vi "Write ID.vi"(8 "id":u32, 11 "Channel Message in":refnum<class "Channel Message.lvclass">) -> (3 "Channel Message out":refnum<class "Channel Message.lvclass">)   [LabVIEW 2017, in "Channel Message.lvclass"]
doc: "Writes the ID for this message. This is done automatically when the message is written into the Messenger Channel."
uses:
  <vilib>/ChannelSupport/Channel Message/Channel Message.lvclass
  <vilib>/ChannelSupport/Channel Message/Channel Message.lvclass/Channel Message.ctl
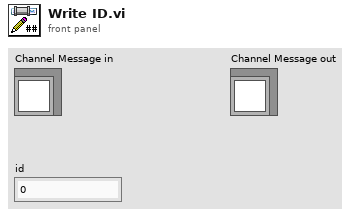
[diagram p1: front panel]
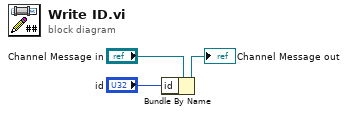
[diagram p0: block diagram]
diagram:
  n1 = Bundle By Name(cluster="Channel Message in", "id"="id") -> (→"Channel Message out":refnum<class "Channel Message.lvclass">)
